vi "VP_Host_Test.vi"() -> ()   [LabVIEW 2015]
uses:
  UI states.ctl
  <vilib>/WebDAVClient/Advanced/Get File.vi
  <vilib>/Utility/config.llb/Write Key (Boolean).vi
  <vilib>/WebDAVClient/Advanced/Put File.vi
  <resource>/objmgr/ni.dex.rc
  <vilib>/nisyscfg/nisyscfg.lvlib
  <resource>/objmgr/nisysapi.rc
  <vilib>/WebDAVClient/NI_WebDAV.lvlib
  <vilib>/Utility/config.llb/NI_LVConfig.lvlib
panel:
  out "Monitor Status":string
  in  "Turn on startup Apps":bool
  in  "Reconnect cRIO":bool
  out "Primary Disk Free (GB)":dbl format="%#_4g"
  out "Primary Disk Capacity (GB)":dbl format="%#_4g"
  out "Free Virtual Memory (GB)":dbl format="%#_4g"
  out "Total Virtual Memory (GB)":dbl format="%#_4g"
  out "Free Physical Memory (GB)":dbl format="%#_4g"
  out "Total Physical Memory (GB)":dbl format="%#_4g"
  out "cRIO System Status":string
  in  "Reboot cRIO":bool
  in  "Target (localhost)":refnum<k21>="localhost"
  in  "Data Loop Period":u32
  out "Velociprobe cRIO error log":string
  in  "Stop Monitor":bool
  in  "Target IP Address":string="localhost"
  out "XY Ref":cluster{dbl[], dbl[]}[](graph)
  out "Reference and Actual positions":cluster{"t0":dbl, dbl, dbl[][]}(graph)
  out "Data Read Period (sec)":dbl=3.9999999999999996e-05
  out "Data Read Rate (Hz)":dbl=25000.000000000004
  out "File plotter loop iterations":i32
  out "Queue is empty":bool=TRUE
  out "Data Frequency":fxp<+,32,0>
  out "Available Elements to Read":i32
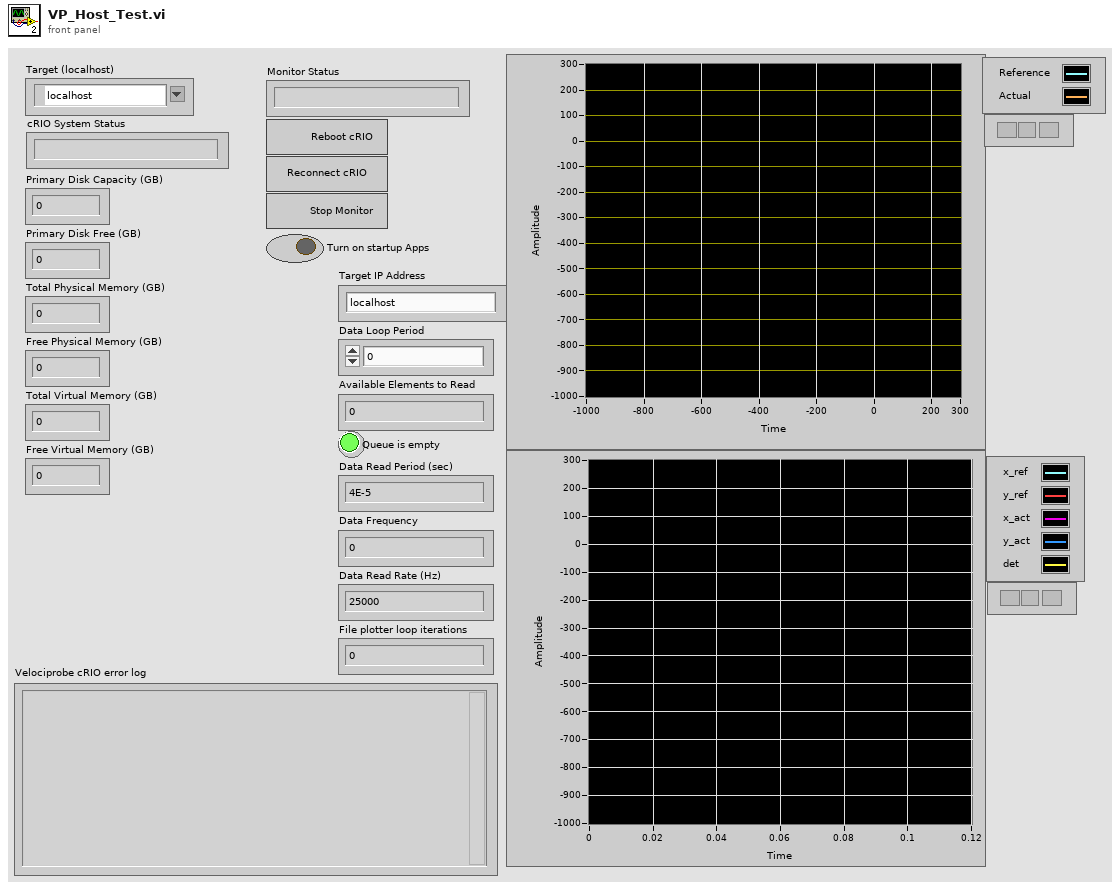
[diagram p1: front panel]
types:
  T1 = typedef "UI states.ctl" = enum16{"Initialize", "Wait", "Turn off cRIO controls "}
  T2 = typedef "NI_WebDAV.lvlib/SessionHandle.ctl" = refnum<k1>
  T3 = typedef "NI_LVConfig.lvlib/Config Data RefNum.ctl" = refnum<k1>
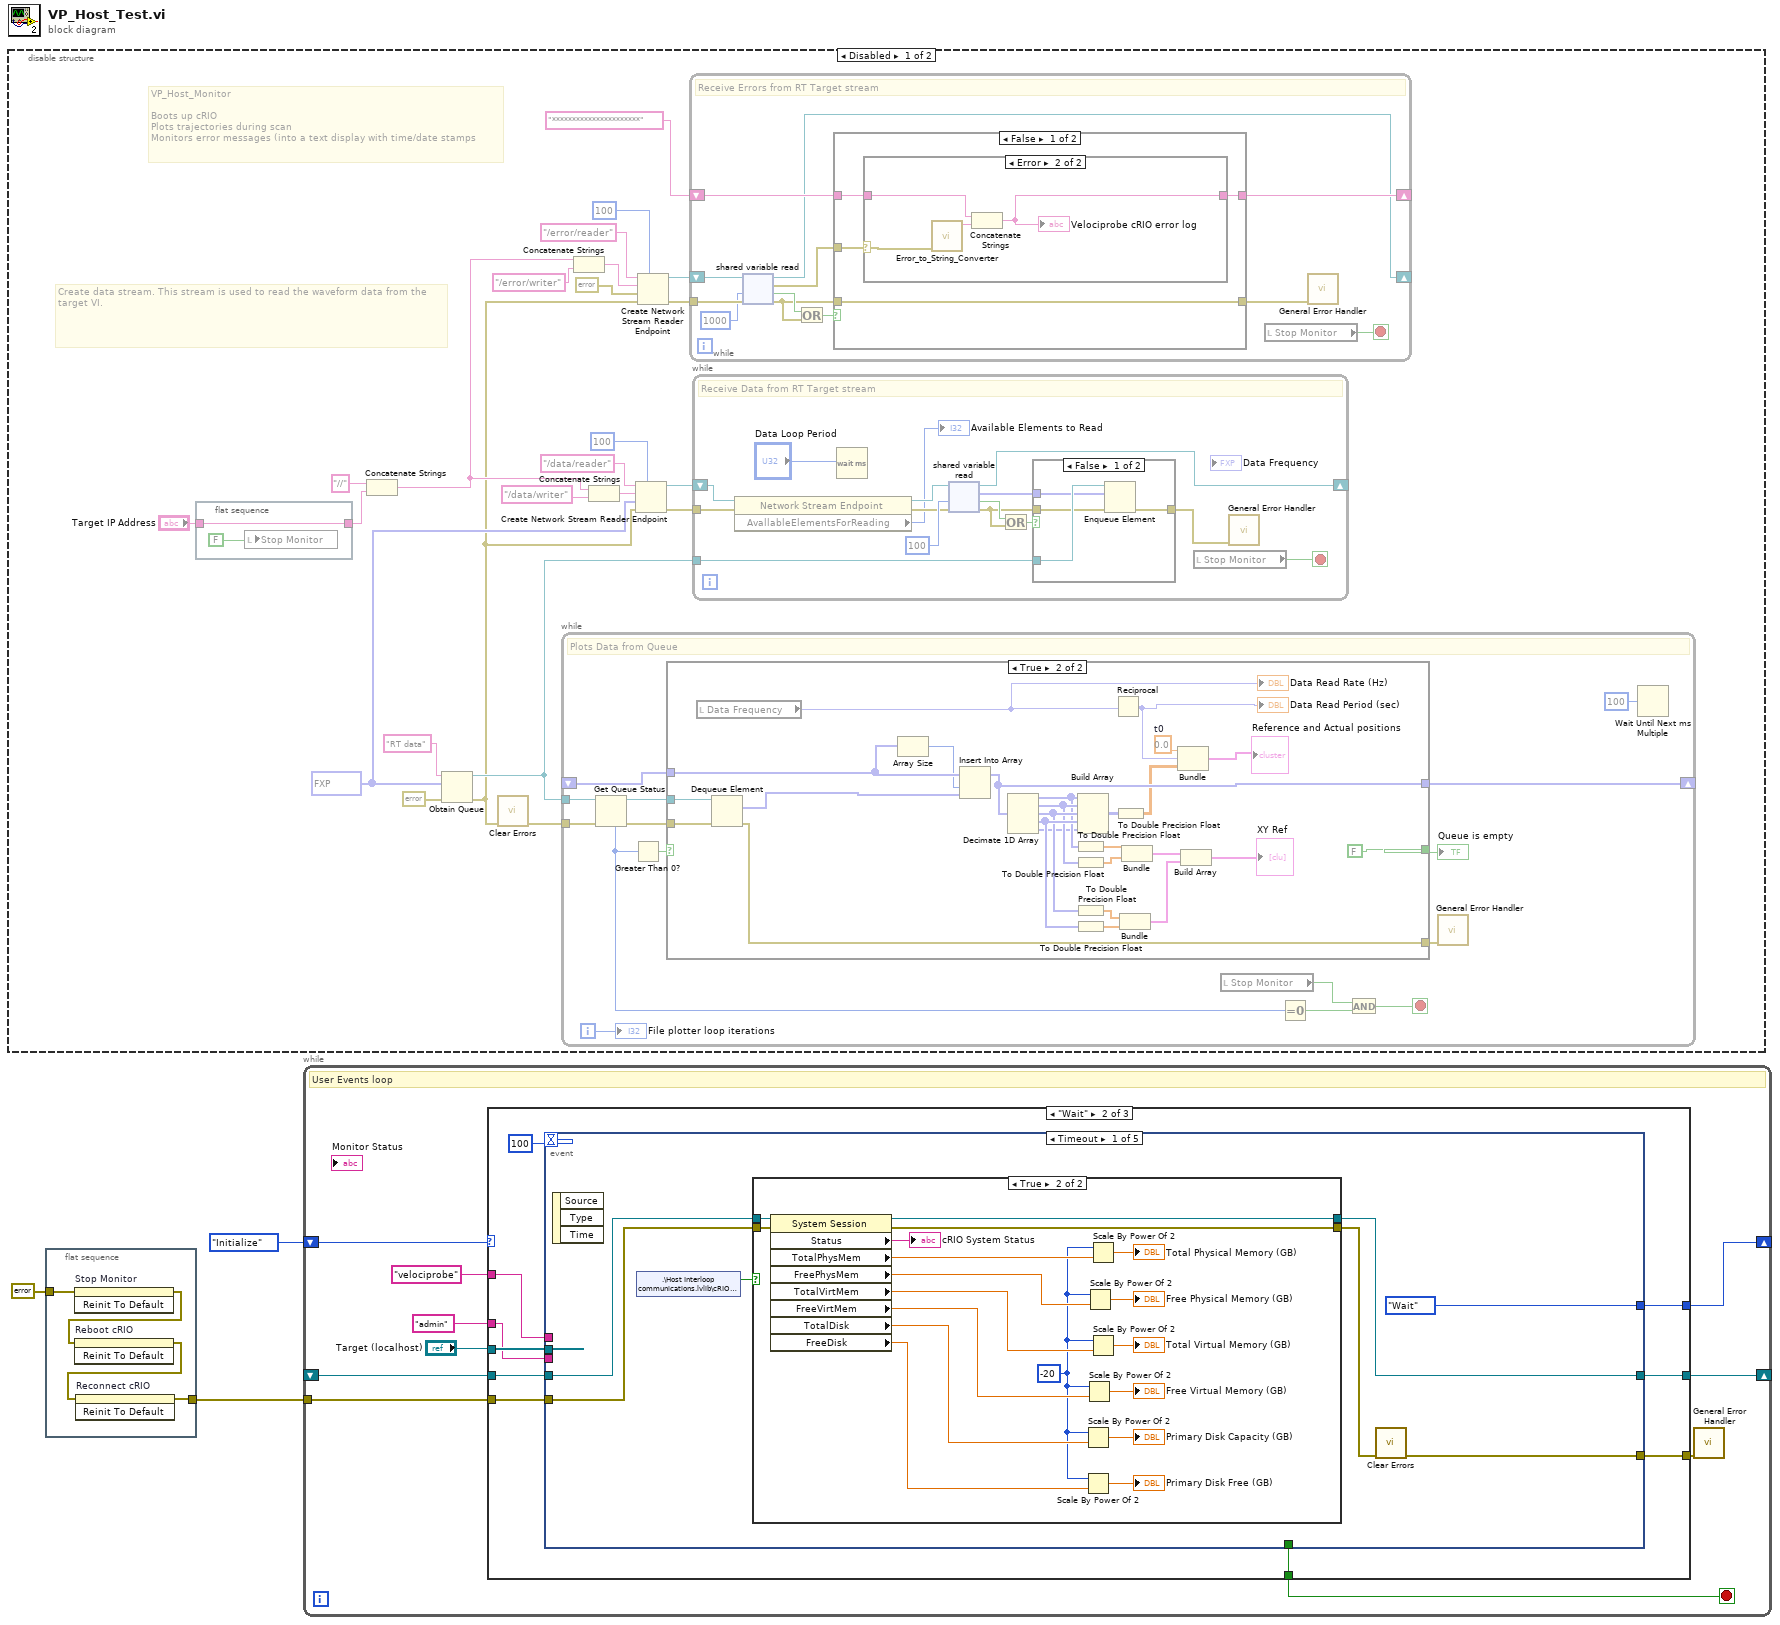
[diagram p0: block diagram]
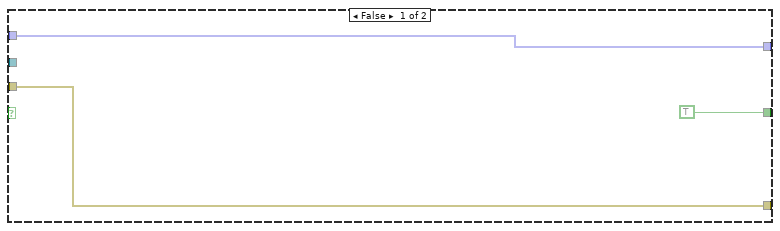
[diagram p4: hidden frame]
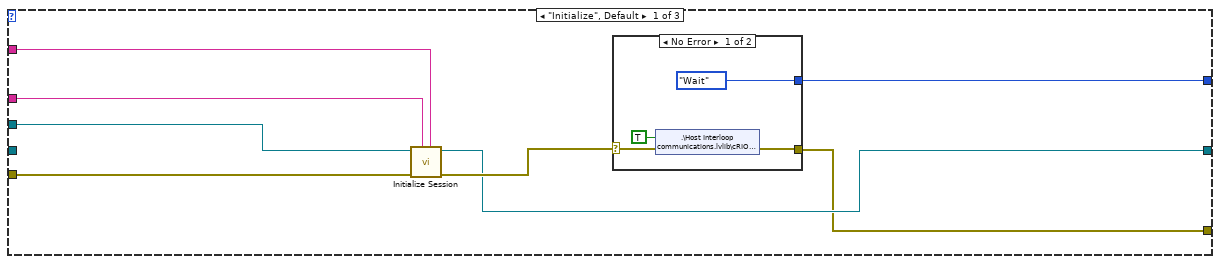
[diagram p7: hidden frame]
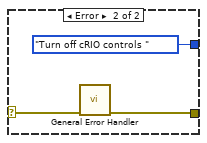
[diagram p8: hidden frame]
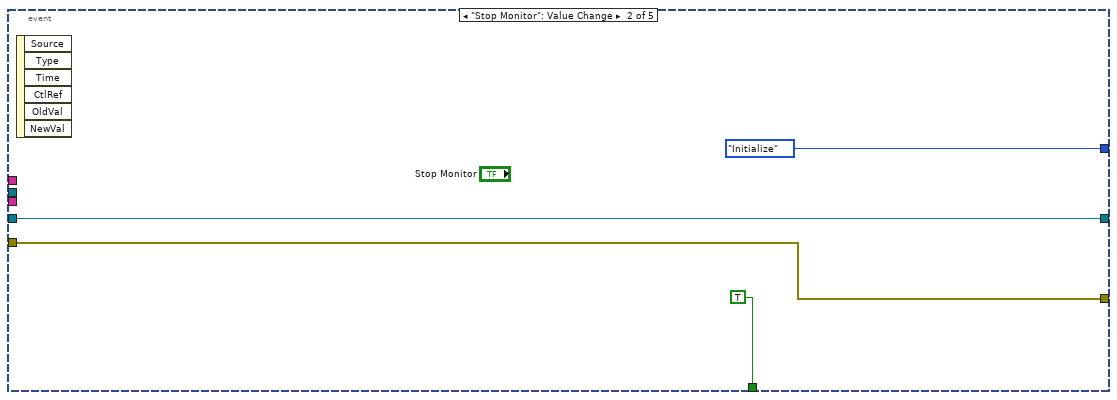
[diagram p10: hidden frame]
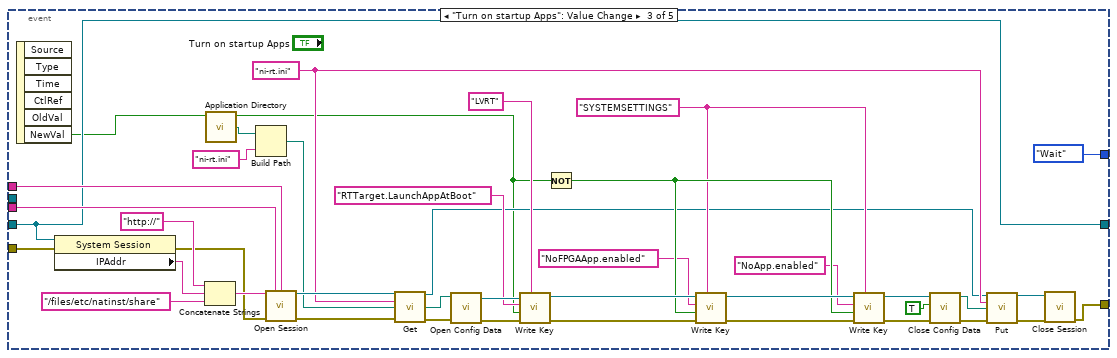
[diagram p11: hidden frame]
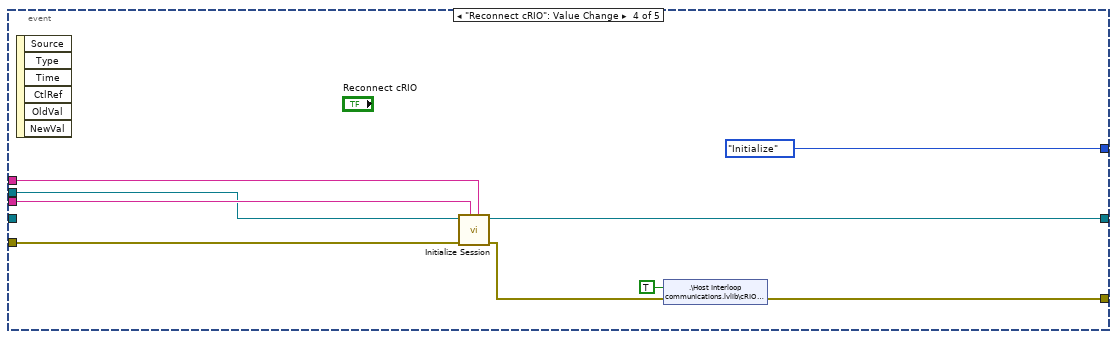
[diagram p12: hidden frame]
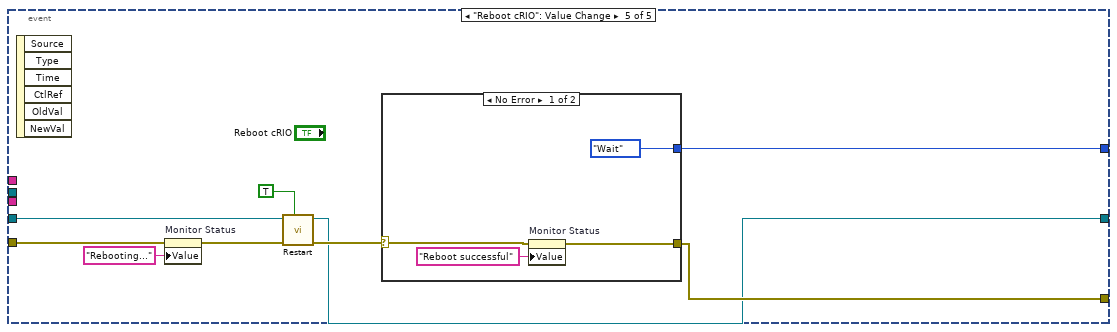
[diagram p13: hidden frame]
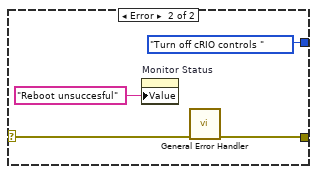
[diagram p14: hidden frame]
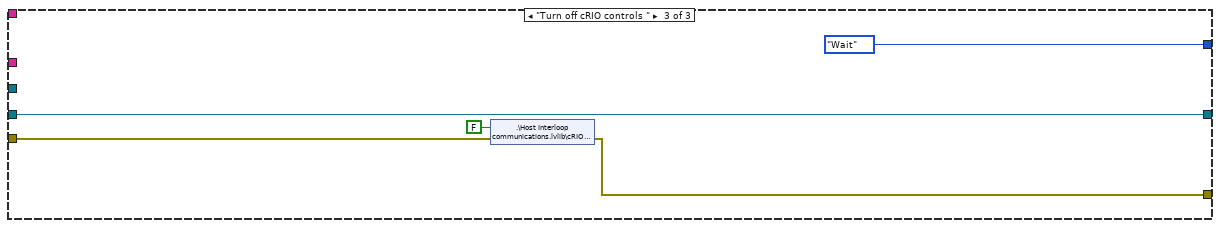
[diagram p15: hidden frame]
diagram:
  n1 = disable-structure shown="Disabled" {
    frame Disabled {
      w16 = fxp<+/-,58,25>[] [0.0, 0.0, 0.0, 0.0, 0.0, 0.0, 0.0, 0.0, 0.0, 0.0, 0.0, 0.0, 0.0, 0.0, 0.0, 0.0, 0.0, 0.0, 0.0, 0.0, 0.0, 0.0, 0.0, 0.0, 0.0, 0.0, 0.0, 0.0, 0.0, 0.0, 0.0, 0.0, 0.0, 0.0, 0.0, 0.0, 0.0, 0.0, 0.0, 0.0, 0.0, 0.0, 0.0, 0.0, 0.0, 0.0, 0.0, 0.0, 0.0, 0.0, 0.0, 0.0, 0.0, 0.0, 0.0, 0.0, 0.0, 0.0, 0.0, 0.0, 0.0, 0.0, 0.0, 0.0, 0.0, 0.0, 0.0, 0.0, 0.0, 0.0, 0.0, 0.0, 0.0, 0.0, 0.0, 0.0, 0.0, 0.0, 0.0, 0.0, 0.0, 0.0, 0.0, 0.0, 0.0, 0.0, 0.0, 0.0, 0.0, 0.0, 0.0, 0.0, 0.0, 0.0, 0.0, 0.0, 0.0, 0.0, 0.0, 0.0, 0.0, 0.0, 0.0, 0.0, 0.0, 0.0, 0.0, 0.0, 0.0, 0.0, 0.0, 0.0, 0.0, 0.0, 0.0, 0.0, 0.0, 0.0, 0.0, 0.0, 0.0, 0.0, 0.0, 0.0, 0.0, 0.0, 0.0, 0.0, 0.0, 0.0, 0.0, 0.0, 0.0, 0.0, 0.0, 0.0, 0.0, 0.0, 0.0, 0.0, 0.0, 0.0, 0.0, 0.0, 0.0, 0.0, 0.0, 0.0, 0.0, 0.0, 0.0, 0.0, 0.0, 0.0, 0.0, 0.0, 0.0, 0.0, 0.0, 0.0, 0.0, 0.0, 0.0, 0.0, 0.0, 0.0, 0.0, 0.0, 0.0, 0.0, 0.0, 0.0, 0.0, 0.0, 0.0, 0.0, 0.0, 0.0, 0.0, 0.0, 0.0, 0.0, 0.0, 0.0, 0.0, 0.0, 0.0, 0.0, 0.0, 0.0, 0.0, 0.0, 0.0, 0.0, 0.0, 0.0, 0.0, 0.0, 0.0, 0.0, 0.0, 0.0, 0.0, 0.0, 0.0, 0.0, 0.0, 0.0, 0.0, 0.0, 0.0, 0.0, 0.0, 0.0, 0.0, 0.0, 0.0, 0.0, 0.0, 0.0, 0.0, 0.0, 0.0, 0.0, 0.0, 0.0, 0.0, 0.0, 0.0, 0.0, 0.0, 0.0, 0.0, 0.0, 0.0, 0.0, 0.0, 0.0, 0.0, 0.0, 0.0, 0.0, 0.0, 0.0, 0.0, 0.0, 0.0, 0.0, 0.0, 0.0, 0.0, 0.0, 0.0, 0.0, 0.0, 0.0, 0.0, 0.0, 0.0, 0.0, 0.0, 0.0, 0.0, 0.0, 0.0, 0.0, 0.0, 0.0, 0.0, 0.0, 0.0, 0.0, 0.0, 0.0, 0.0, 0.0, 0.0, 0.0, 0.0, 0.0, 0.0, 0.0, 0.0, 0.0, 0.0, 0.0, 0.0, 0.0, 0.0, 0.0, 0.0, 0.0, 0.0, 0.0, 0.0, 0.0, 0.0, 0.0, 0.0, 0.0, 0.0, 0.0, 0.0, 0.0, 0.0, 0.0, 0.0, 0.0, 0.0, 0.0, 0.0, 0.0, 0.0, 0.0, 0.0, 0.0, 0.0, 0.0, 0.0, 0.0, 0.0, 0.0, 0.0, 0.0, 0.0, 0.0, 0.0, 0.0, 0.0, 0.0, 0.0, 0.0, 0.0, 0.0, 0.0, 0.0, 0.0, 0.0, 0.0, 0.0, 0.0, 0.0, 0.0, 0.0, 0.0, 0.0, 0.0, 0.0, 0.0, 0.0, 0.0, 0.0, 0.0, 0.0, 0.0, 0.0, 0.0, 0.0, 0.0, 0.0, 0.0, 0.0, 0.0, 0.0, 0.0, 0.0, 0.0, 0.0, 0.0, 0.0, 0.0, 0.0, 0.0, 0.0, 0.0, 0.0, 0.0, 0.0, 0.0, 0.0, 0.0, 0.0, 0.0, 0.0, 0.0, 0.0, 0.0, 0.0, 0.0, 0.0, 0.0, 0.0, 0.0, 0.0, 0.0, 0.0, 0.0, 0.0, 0.0, 0.0, 0.0, 0.0, 0.0, 0.0, 0.0, 0.0, 0.0, 0.0, 0.0, 0.0, 0.0, 0.0, 0.0, 0.0, 0.0, 0.0, 0.0, 0.0, 0.0, 0.0, 0.0, 0.0, 0.0, 0.0, 0.0, 0.0, 0.0, 0.0, 0.0, 0.0, 0.0, 0.0, 0.0, 0.0, 0.0, 0.0, 0.0, 0.0, 0.0, 0.0, 0.0, 0.0, 0.0, 0.0, 0.0, 0.0, 0.0, 0.0, 0.0, 0.0, 0.0, 0.0, 0.0, 0.0, 0.0, 0.0, 0.0, 0.0, 0.0, 0.0, 0.0, 0.0, 0.0, 0.0, 0.0, 0.0, 0.0, 0.0, 0.0, 0.0, 0.0, 0.0, 0.0, 0.0, 0.0, 0.0, 0.0, 0.0, 0.0, 0.0, 0.0, 0.0, 0.0, 0.0, 0.0, 0.0, 0.0, 0.0, 0.0, 0.0, 0.0, 0.0, 0.0, 0.0, 0.0, 0.0, 0.0, 0.0, 0.0, 0.0, 0.0, 0.0, 0.0, 0.0, 0.0, 0.0, 0.0, 0.0, 0.0, 0.0, 0.0, 0.0, 0.0, 0.0, 0.0, 0.0, 0.0, 0.0, 0.0, 0.0, 0.0, 0.0, 0.0, 0.0, 0.0, 0.0, 0.0, 0.0, 0.0, 0.0, 0.0, 0.0, 0.0, 0.0, 0.0, 0.0, 0.0, 0.0, 0.0, 0.0, 0.0, 0.0, 0.0, 0.0, 0.0, 0.0, 0.0, 0.0, 0.0, 0.0, 0.0, 0.0, 0.0, 0.0, 0.0, 0.0, 0.0, 0.0, 0.0, 0.0, 0.0, 0.0, 0.0, 0.0, 0.0, 0.0, 0.0, 0.0, 0.0, 0.0, 0.0, 0.0, 0.0, 0.0, 0.0, 0.0, 0.0, 0.0, 0.0, 0.0, 0.0, 0.0, 0.0, 0.0, 0.0, 0.0, 0.0, 0.0, 0.0, 0.0, 0.0, 0.0, 0.0, 0.0, 0.0, 0.0, 0.0, 0.0, 0.0, 0.0, 0.0, 0.0, 0.0, 0.0, 0.0, 0.0, 0.0, 0.0, 0.0, 0.0, 0.0, 0.0, 0.0, 0.0, 0.0, 0.0, 0.0, 0.0, 0.0, 0.0, 0.0, 0.0, 0.0, 0.0, 0.0, 0.0, 0.0, 0.0, 0.0, 0.0, 0.0, 0.0, 0.0, 0.0, 0.0, 0.0, 0.0, 0.0, 0.0, 0.0, 0.0, 0.0, 0.0, 0.0, 0.0, 0.0, 0.0, 0.0, 0.0, 0.0, 0.0, 0.0, 0.0, 0.0, 0.0, 0.0, 0.0, 0.0, 0.0, 0.0, 0.0, 0.0, 0.0, 0.0, 0.0, 0.0, 0.0, 0.0, 0.0, 0.0, 0.0, 0.0, 0.0, 0.0, 0.0, 0.0, 0.0, 0.0, 0.0, 0.0, 0.0, 0.0, 0.0, 0.0, 0.0, 0.0, 0.0, 0.0, 0.0, 0.0, 0.0, 0.0, 0.0, 0.0, 0.0, 0.0, 0.0, 0.0, 0.0, 0.0, 0.0, 0.0, 0.0, 0.0, 0.0, 0.0, 0.0, 0.0, 0.0, 0.0, 0.0, 0.0, 0.0, 0.0, 0.0, 0.0, 0.0, 0.0, 0.0, 0.0, 0.0, 0.0, 0.0, 0.0, 0.0, 0.0, 0.0, 0.0, 0.0, 0.0, 0.0, 0.0, 0.0, 0.0, 0.0, 0.0, 0.0, 0.0, 0.0, 0.0, 0.0, 0.0, 0.0, 0.0, 0.0, 0.0, 0.0, 0.0, 0.0, 0.0, 0.0, 0.0, 0.0, 0.0, 0.0, 0.0, 0.0, 0.0, 0.0, 0.0, 0.0, 0.0, 0.0, 0.0, 0.0, 0.0, 0.0, 0.0, 0.0, 0.0, 0.0, 0.0, 0.0, 0.0, 0.0, 0.0, 0.0, 0.0, 0.0, 0.0, 0.0, 0.0, 0.0, 0.0, 0.0, 0.0, 0.0, 0.0, 0.0, 0.0, 0.0, 0.0, 0.0, 0.0, 0.0, 0.0, 0.0, 0.0, 0.0, 0.0, 0.0, 0.0, 0.0, 0.0, 0.0, 0.0, 0.0, 0.0, 0.0, 0.0, 0.0, 0.0, 0.0, 0.0, 0.0, 0.0, 0.0, 0.0, 0.0, 0.0, 0.0, 0.0, 0.0, 0.0, 0.0, 0.0, 0.0, 0.0, 0.0, 0.0, 0.0, 0.0, 0.0, 0.0, 0.0, 0.0, 0.0, 0.0, 0.0, 0.0, 0.0, 0.0, 0.0, 0.0, 0.0, 0.0, 0.0, 0.0, 0.0, 0.0, 0.0, 0.0, 0.0, 0.0, 0.0, 0.0, 0.0, 0.0, 0.0, 0.0, 0.0, 0.0, 0.0, 0.0, 0.0, 0.0, 0.0, 0.0, 0.0, 0.0, 0.0, 0.0, 0.0, 0.0, 0.0, 0.0, 0.0, 0.0, 0.0, 0.0, 0.0, 0.0, 0.0, 0.0, 0.0, 0.0, 0.0, 0.0, 0.0, 0.0, 0.0, 0.0, 0.0, 0.0, 0.0, 0.0, 0.0, 0.0, 0.0, 0.0, 0.0, 0.0, 0.0, 0.0, 0.0, 0.0, 0.0, 0.0, 0.0, 0.0, 0.0, 0.0, 0.0, 0.0, 0.0, 0.0, 0.0, 0.0, 0.0, 0.0, 0.0, 0.0, 0.0, 0.0, 0.0, 0.0, 0.0, 0.0, 0.0, 0.0, 0.0, 0.0, 0.0, 0.0, 0.0, 0.0, 0.0, 0.0, 0.0, 0.0, 0.0, 0.0, 0.0, 0.0, 0.0, 0.0, 0.0, 0.0, 0.0, 0.0, 0.0, 0.0, 0.0, 0.0, 0.0, 0.0, 0.0, 0.0, 0.0, 0.0, 0.0, 0.0, 0.0, 0.0, 0.0, 0.0, 0.0, 0.0, 0.0, 0.0, 0.0, 0.0, 0.0, 0.0, 0.0, 0.0, 0.0, 0.0, 0.0, 0.0, 0.0, 0.0, 0.0, 0.0, 0.0, 0.0, 0.0, 0.0, 0.0, 0.0, 0.0, 0.0, 0.0, 0.0, 0.0, 0.0, 0.0, 0.0, 0.0, 0.0, 0.0, 0.0, 0.0, 0.0, 0.0, 0.0, 0.0, 0.0, 0.0, 0.0, 0.0, 0.0, 0.0, 0.0, 0.0, 0.0, 0.0, 0.0, 0.0, 0.0, 0.0, 0.0, 0.0, 0.0, 0.0, 0.0, 0.0, 0.0, 0.0, 0.0, 0.0, 0.0, 0.0, 0.0, 0.0, 0.0, 0.0, 0.0, 0.0, 0.0, 0.0, 0.0, 0.0, 0.0, 0.0, 0.0, 0.0, 0.0, 0.0, 0.0, 0.0, 0.0, 0.0, 0.0, 0.0, 0.0, 0.0, 0.0, 0.0, 0.0, 0.0, 0.0, 0.0, 0.0, 0.0, 0.0, 0.0, 0.0, 0.0, 0.0, 0.0, 0.0, 0.0, 0.0, 0.0, 0.0, 0.0, 0.0, 0.0, 0.0, 0.0, 0.0, 0.0, 0.0, 0.0, 0.0, 0.0, 0.0, 0.0, 0.0, 0.0, 0.0, 0.0, 0.0, 0.0, 0.0, 0.0, 0.0, 0.0, 0.0, 0.0, 0.0, 0.0, 0.0, 0.0, 0.0, 0.0, 0.0, 0.0, 0.0, 0.0, 0.0, 0.0, 0.0, 0.0, 0.0, 0.0, 0.0, 0.0, 0.0, 0.0, 0.0, 0.0, 0.0, 0.0, 0.0, 0.0, 0.0, 0.0, 0.0, 0.0, 0.0, 0.0, 0.0, 0.0, 0.0, 0.0, 0.0, 0.0, 0.0, 0.0, 0.0, 0.0, 0.0, 0.0, 0.0, 0.0, 0.0, 0.0, 0.0, 0.0, 0.0, 0.0, 0.0, 0.0, 0.0, 0.0, 0.0, 0.0, 0.0, 0.0, 0.0, 0.0, 0.0, 0.0, 0.0, 0.0, 0.0, 0.0, 0.0, 0.0, 0.0, 0.0, 0.0, 0.0, 0.0, 0.0, 0.0, 0.0, 0.0, 0.0, 0.0, 0.0, 0.0, 0.0, 0.0, 0.0, 0.0, 0.0, 0.0, 0.0, 0.0, 0.0, 0.0, 0.0, 0.0, 0.0, 0.0, 0.0, 0.0, 0.0, 0.0, 0.0, 0.0, 0.0, 0.0, 0.0, 0.0, 0.0, 0.0, 0.0, 0.0, 0.0, 0.0, 0.0, 0.0, 0.0, 0.0, 0.0, 0.0, 0.0, 0.0, 0.0, 0.0, 0.0, 0.0, 0.0, 0.0, 0.0, 0.0, 0.0, 0.0, 0.0, 0.0, 0.0, 0.0, 0.0, 0.0, 0.0, 0.0, 0.0, 0.0, 0.0, 0.0, 0.0, 0.0, 0.0, 0.0, 0.0, 0.0] ("Data 2")
      # "VP_Host_Monitor\n\nBoots up cRIO\nPlots trajectories during scan\nMonitors error messages (into a text display with time/date stamps"
      # "Create data stream. This stream is used to read the waveform data from the target VI."
      n2 = flat-sequence {
        tunnel: "Target IP Address" -> [w52]
        tunnel: [w52] -> w17
        frame #0 {
          n3 = local write "Stop Monitor"(FALSE ("Host Stop")) -> ()
        }
      }
      n4 = Concatenate Strings("//" ("reader url"), w17) -> (w10:string)
      n5 = Obtain Queue(name (unnamed)="RT data", element data type=w16, error in (no error)=errorcluster {"status"=FALSE, "code"=0, "source"=""}) -> (queue out=w26:refnum<queue>, error out=w8:errorcluster)  [unwired: 2 in, 1 out]
      n6 = call <vilib>:"Clear Errors.vi"("error in (no error)"=w8) -> ("error out"=w27:errorcluster)  [unwired: 5 in, 1 out]
      n7 = while {
        tunnel: w26 -> [w67]
        shift-right: [w57] -> _
        shift-left: _ -> [w56]
        tunnel: w27 -> [w66]
        i -> [w59]
        stop <- w60 stop-if-true
        # "Plots Data from Queue"
        n8 = Get Queue Status(queue=w67, error in (no error)=w66) -> (queue out=w64:refnum<queue>, error out=w65:errorcluster, # elements in queue=w62:i32)  [unwired: 1 in, 5 out]
        n9 = Greater Than 0?(x=w62) -> (x > 0?=w63:bool)
        n10 = case shown="True" w63 {
          tunnel: w65 -> [w69 w96]
          tunnel: w64 -> [_ w95]
          tunnel: [w69 w86] -> w53
          tunnel: [TRUE FALSE] -> w58
          tunnel: [w68 w93] -> w57
          tunnel: w56 -> [w68 w92]
          frame False {
          }
          frame True {
            w79 = 0.0  # t0
            n11 = local read "Data Frequency"() -> (w87:fxp<+,32,0>)
            "Data Read Rate (Hz)" <- w87
            n12 = Dequeue Element(queue=w95, error in (no error)=w96) -> (element=w91:fxp<+/-,58,25>[], error out=w86:errorcluster)  [unwired: 1 in, 2 out]
            n13 = Array Size(array=w92) -> (size(s)=w73:i32)
            n14 = Insert Into Array(array=w92, index=w73, new element=w91) -> (w93:fxp<+/-,58,25>[])
            n15 = Decimate 1D Array(w93) -> (w82:fxp<+/-,58,25>[], w83:fxp<+/-,58,25>[], w84:fxp<+/-,58,25>[], w85:fxp<+/-,58,25>[], w81:fxp<+/-,58,25>[])
            n16 = To Double Precision Float(number=w82) -> (double precision float=w77:dbl[])
            n17 = To Double Precision Float(number=w83) -> (double precision float=w76:dbl[])
            n18 = To Double Precision Float(number=w84) -> (double precision float=w75:dbl[])
            n19 = To Double Precision Float(number=w85) -> (double precision float=w74:dbl[])
            n20 = Build Array(w82, w83, w84, w85, w81) -> (w80:fxp<+/-,58,25>[][])
            n21 = Reciprocal(x=w87) -> (1/x=w88:fxp<+,33,33>)
            "Data Read Period (sec)" <- w88
            n22 = To Double Precision Float(number=w80) -> (double precision float=w71:dbl[][])
            n23 = Bundle(w75, w74) -> (w72:cluster{dbl[], dbl[]})  [unwired: 1 in]
            n24 = Bundle(w77, w76) -> (w78:cluster{dbl[], dbl[]})  [unwired: 1 in]
            n25 = Bundle("t0"=w79, w88, w71) -> (→"Reference and Actual positions":cluster{"t0":dbl, fxp<+,33,33>, dbl[][]})  [unwired: 1 in]
            n26 = Build Array(w78, w72) -> (→"XY Ref":cluster{dbl[], dbl[]}[])
          }
        }
        "Queue is empty" <- w58
        n27 = local read "Stop Monitor"() -> (w54:bool)
        n28 = Equal To 0?(x=w62) -> (x = 0?=w61:bool)
        n29 = And(x=w54, y=w61) -> (x .and. y?=w60:bool)
        n30 = call <vilib>:"General Error Handler.vi"("error in (no error)"=w53) -> ()  [unwired: 10 in, 5 out]
        n31 = Wait Until Next ms Multiple(millisecond multiple=u32 100) -> ()  [unwired: 1 out]
        "File plotter loop iterations" <- w59
      }
      n32 = Concatenate Strings(w10, "/error/writer" ("reader url")) -> (w13:string)
      n33 = Concatenate Strings(w10, "/data/writer" ("reader url")) -> (w20:string)
      n34 = Create Network Stream Reader Endpoint(7:100 ("reader buffer size"), 8:w8, 9:w16, 10:w20, 11:"/data/reader" ("writer name")) -> (0:w9:errorcluster, 3:w15:refnum<k21>)  [unwired: 2 in]
      n35 = Create Network Stream Reader Endpoint(7:100 ("reader buffer size"), 8:w8, 9:errorcluster {"status"=FALSE, "code"=0, "source"=""} ("error constant"), 10:w13, 11:"/error/reader" ("writer name")) -> (0:w5:errorcluster, 3:w6:refnum<k21>)  [unwired: 2 in]
      n36 = while "Host->Target Command Reader" {
        shift-right: [w29] -> _
        shift-left: w6 -> [w38]
        shift-right: [w31] -> _
        shift-left: "**********************" -> [w30]
        tunnel: w5 -> [w39]
        stop <- w32 stop-if-true
        # "Receive Errors from RT Target stream"
        n37 = shared-variable-read(w38, w39, 1000 ("timeout ms")) -> (w29:refnum<k21>, w33:errorcluster, w35:bool, w36:errorcluster)
        n38 = Or(x=w35, y=w33) -> (x .or. y?=w34:bool)
        n39 = case shown="False" w34 {
          tunnel: w33 -> [w43 w50]
          tunnel: [w43 w50] -> w28
          tunnel: w36 -> [w40 _]
          tunnel: [w42 w49] -> w31
          tunnel: w30 -> [w41 w49]
          frame False {
            n40 = case shown="Error" w40 {
              selector: w40 -> [_ w48]
              tunnel: [w44 w46] -> w42
              tunnel: w41 -> [w44 w45]
              frame No Error {
              }
              frame Error {
                n41 = call "Error_to_String_Converter.vi"("error in"=w48) -> ("String"=w47:string)  [unwired: 9 in, 1 out]
                n42 = Concatenate Strings(w45, w47) -> (w46:string)
                "Velociprobe cRIO error log" <- w46
              }
            }
          }
          frame True {
          }
        }
        n43 = local read "Stop Monitor"() -> (w32:bool)
        n44 = call <vilib>:"General Error Handler.vi"("error in (no error)"=w28) -> ()  [unwired: 10 in, 5 out]
      }
      n45 = while "Target->Host Data Reader" {
        shift-right: [w108] -> _
        shift-left: w15 -> [w105]
        tunnel: w26 -> [w100]
        tunnel: w9 -> [w103]
        stop <- w99 stop-if-true
        # "Receive Data from RT Target stream"
        n46 = property class="Network Stream Endpoint"(reference=w105, error in=w103) -> (reference out=w104:refnum<k21>, error out=w102:errorcluster, "AvallableElementsForReading"=→"Available Elements to Read":i32)
        n47 = Wait (ms)(milliseconds to wait="Data Loop Period") -> ()  [unwired: 1 out]
        n48 = shared-variable-read(w104, w102, 100 ("timeout ms")) -> (w108:refnum<k21>, w107:errorcluster, w110:bool, w111:fxp<+/-,58,25>[])
        n49 = Or(x=w110, y=w107) -> (x .or. y?=w109:bool)
        n50 = case shown="False" w109 {
          tunnel: w111 -> [w114 _]
          tunnel: w107 -> [w113 w116]
          tunnel: [w112 w116] -> w97
          tunnel: w100 -> [w115 _]
          frame False {
            n51 = Enqueue Element(queue=w115, element=w114, error in (no error)=w113) -> (error out=w112:errorcluster)  [unwired: 1 in, 2 out]
          }
          frame True {
          }
        }
        n52 = local read "Stop Monitor"() -> (w99:bool)
        n53 = call <vilib>:"General Error Handler.vi"("error in (no error)"=w97) -> ()  [unwired: 10 in, 5 out]
      }
    }
    frame Enabled {
    }
  }
  n54 = flat-sequence {
    tunnel: errorcluster {"status"=FALSE, "code"=0, "source"=""} ("error in (no error)") -> [w118]
    tunnel: [w117] -> w1
    frame #0 {
      n55 = invoke on="Stop Monitor" class="Bool" method="Reinit To Default"(error in=w118) -> (error out=w120:errorcluster)  [unwired: 2 in, 2 out]
      n56 = invoke on="Reboot cRIO" class="Bool" method="Reinit To Default"(error in=w120) -> (error out=w119:errorcluster)  [unwired: 2 in, 2 out]
      n57 = invoke on="Reconnect cRIO" class="Bool" method="Reinit To Default"(error in=w119) -> (error out=w117:errorcluster)  [unwired: 2 in, 2 out]
    }
  }
  n58 = while {
    tunnel: w1 -> [w128]
    shift-right: [w126] -> _
    shift-left: UI_states."Initialize" -> [w127]
    shift-right: [w125] -> _
    shift-left: _ -> [w129]
    stop <- w130 stop-if-true
    # "User Events loop"
    n59 = case shown="\"Wait\"" w127 {
      tunnel: [_ w155 _] -> w130
      tunnel: w129 -> [_ w153 w253]
      tunnel: w128 -> [w136 w152 w254]
      tunnel: [w135 w151 UI_states."Wait"] -> w126
      tunnel: [w137 w149 w253] -> w125
      tunnel: [w134 w150 w255] -> w124
      tunnel: "Target (localhost)" -> [w133 w146 _]
      tunnel: "velociprobe" ("Password") -> [w132 w147 _]
      tunnel: "admin" ("User Name") -> [w131 w148 _]
      frame "Initialize", Default {
        n60 = call <vilib>:"Initialize Session.vi"("Password"=w132, "User Name"=w131, "error in (no error)"=w136, "Target (localhost)"=w133) -> ("error out"=w138:errorcluster, "Session out"=w137:refnum<k21>)  [unwired: 6 in]
        n61 = case shown="No Error" w138 {
          selector: w138 -> [w141 w144]
          tunnel: [UI_states."Wait" UI_states."Turn off cRIO controls "] -> w135
          tunnel: [w140 w143] -> w134
          frame No Error {
            n62 = shared-variable ".\\Host Interloop communications.lvlib\\cRIO status"(TRUE ("cRIO status"), error in=w141) -> (error out=w140:errorcluster)
          }
          frame Error {
            n63 = call <vilib>:"General Error Handler.vi"("error in (no error)"=w144) -> ("error out"=w143:errorcluster)  [unwired: 10 in, 4 out]
          }
        }
      }
      frame "Wait" {
        n64 = event shown="[0] Timeout" {
          selector: _ -> [_ _ _ _ _]
          dyn-events: _ -> [_ _ _ _ _]
          timeout: 100 -> [_ _ _ _ _]
          tunnel: [_ TRUE _ _ _] -> w155
          tunnel: w153 -> [w162 w183 w188 _ w244]
          tunnel: w152 -> [w161 w184 w226 w233 w237]
          tunnel: [UI_states."Wait" UI_states."Initialize" UI_states."Wait" UI_states."Initialize" w243] -> w151
          tunnel: [w156 w184 w210 w228 w241] -> w150
          tunnel: [w157 w183 w188 w234 w240] -> w149
          tunnel: w148 -> [_ _ w190 w232 _]
          tunnel: w147 -> [_ _ w189 w231 _]
          tunnel: w146 -> [_ _ _ w230 _]
          event Timeout {
            n65 = event-data() -> ()  [unwired: 1 in, 3 out]
            n66 = shared-variable ".\\Host Interloop communications.lvlib\\cRIO status"() -> (w159:bool)  [unwired: 1 in, 1 out]
            n67 = case shown="True" w159 {
              tunnel: w162 -> [w163 w182]
              tunnel: w161 -> [w164 w181]
              tunnel: [w164 w174] -> w158
              tunnel: [w163 w173] -> w157
              frame False {
              }
              frame True {
                w165 = -20
                n68 = property class="System Session"(reference=w182, error in=w181) -> (reference out=w173:refnum<k21>, error out=w174:errorcluster, "Status"=→"cRIO System Status":string, "TotalPhysMem"=w179:dbl, "FreePhysMem"=w178:dbl, "TotalVirtMem"=w172:dbl, "FreeVirtMem"=w177:dbl, "TotalDisk"=w176:dbl, "FreeDisk"=w175:dbl)
                n69 = Scale By Power Of 2(n=w165, x=w176) -> (x*2^n=→"Primary Disk Capacity (GB)":dbl)
                n70 = Scale By Power Of 2(n=w165, x=w175) -> (x*2^n=→"Primary Disk Free (GB)":dbl)
                n71 = Scale By Power Of 2(n=w165, x=w177) -> (x*2^n=→"Free Virtual Memory (GB)":dbl)
                n72 = Scale By Power Of 2(n=w165, x=w178) -> (x*2^n=→"Free Physical Memory (GB)":dbl)
                n73 = Scale By Power Of 2(n=w165, x=w179) -> (x*2^n=→"Total Physical Memory (GB)":dbl)
                n74 = Scale By Power Of 2(n=w165, x=w172) -> (x*2^n=→"Total Virtual Memory (GB)":dbl)
              }
            }
            n75 = call <vilib>:"Clear Errors.vi"("error in (no error)"=w158) -> ("error out"=w156:errorcluster)  [unwired: 5 in, 1 out]
          }
          event "Stop Monitor": Value Change {
            n76 = event-data() -> ()  [unwired: 1 in, 6 out]
          }
          event "Turn on startup Apps": Value Change {
            w195 = "SYSTEMSETTINGS" ("section")
            w208 = "ni-rt.ini" ("username")
            n77 = event-data() -> ("NewVal"=w187:bool)  [unwired: 1 in, 5 out]
            n78 = property class="System Session"(reference=w188, error in=w226) -> (error out=w221:errorcluster, "IPAddr"=w225:string)  [unwired: 1 out]
            n79 = Concatenate Strings("http://" ("string"), w225, "/files/etc/natinst/share" ("string")) -> (w222:string)
            n80 = call <vilib>:"Application Directory.vi"() -> ("Application Directory"=w216:path)
            n81 = Build Path(base path=w216, name or relative path="ni-rt.ini" ("username")) -> (appended path=w217:path)
            n82 = call <vilib>:"Open Session.vi"("host uri prefix"=w222, "username"=w190, "password"=w189, "error in (no error)"=w221) -> ("session handle out"=w219:T2, "error out"=w220:errorcluster)  [unwired: 10 in]
            n83 = call-poly <vilib>:"Get.vi"("session handle"=w219, "relative uri"=w208, "local file path"=w217, "error in (no error)"=w220) -> ("session handle out"=w192:T2, "local file path out"=w214:path, "error out"=w215:errorcluster)  [unwired: 9 in]
            n84 = call <vilib>:"Open Config Data.vi"("error in (no error)"=w215, "configuration file path"=w214) -> ("error out"=w206:errorcluster, "refnum"=w205:T3)  [unwired: 7 in, 1 out]
            n85 = call-poly <vilib>:"Write Key.vi"("section"="LVRT", "error in (no error)"=w206, "value"=w187, "key"="RTTarget.LaunchAppAtBoot", "refnum"=w205) -> ("error out"=w202:errorcluster, "refnum out"=w199:T3)  [unwired: 4 in, 1 out]
            n86 = Not(x=w187) -> (.not. x?=w196:bool)
            n87 = call-poly <vilib>:"Write Key.vi"("section"=w195, "error in (no error)"=w202, "value"=w196, "key"="NoFPGAApp.enabled", "refnum"=w199) -> ("error out"=w201:errorcluster, "refnum out"=w198:T3)  [unwired: 4 in, 1 out]
            n88 = call-poly <vilib>:"Write Key.vi"("section"=w195, "error in (no error)"=w201, "value"=w196, "key"="NoApp.enabled", "refnum"=w198) -> ("error out"=w200:errorcluster, "refnum out"=w197:T3)  [unwired: 4 in, 1 out]
            n89 = call <vilib>:"Close Config Data.vi"("error in (no error)"=w200, "write file if changed (T)"=TRUE, "refnum"=w197) -> ("error out"=w213:errorcluster, "file path"=w191:path)  [unwired: 7 in]
            n90 = call-poly <vilib>:"Put.vi"("session handle"=w192, "relative uri"=w208, "local file path"=w191, "error in (no error)"=w213) -> ("session handle out"=w212:T2, "error out"=w211:errorcluster)  [unwired: 9 in, 1 out]
            n91 = call <vilib>:"Close Session.vi"("session handle"=w212, "error in (no error)"=w211) -> ("error out"=w210:errorcluster)  [unwired: 13 in]
          }
          event "Reconnect cRIO": Value Change {
            n92 = event-data() -> ()  [unwired: 1 in, 6 out]
            n93 = call <vilib>:"Initialize Session.vi"("Password"=w231, "User Name"=w232, "error in (no error)"=w233, "Target (localhost)"=w230) -> ("error out"=w229:errorcluster, "Session out"=w234:refnum<k21>)  [unwired: 6 in]
            n94 = shared-variable ".\\Host Interloop communications.lvlib\\cRIO status"(TRUE ("cRIO status"), error in=w229) -> (error out=w228:errorcluster)
          }
          event "Reboot cRIO": Value Change {
            n95 = event-data() -> ()  [unwired: 1 in, 6 out]
            n96 = property on="Monitor Status" class="Str"(error in=w237, "Value"="Rebooting..." ("Status")) -> (error out=w238:errorcluster)  [unwired: 1 in, 1 out]
            n97 = call <vilib>:"Restart.vi"("Wait Until Complete (T)"=TRUE, "error in (no error)"=w238, "Session in"=w244) -> ("error out"=w242:errorcluster, "Session out"=w240:refnum<k21>)  [unwired: 6 in, 1 out]
            n98 = case shown="No Error" w242 {
              selector: w242 -> [w246 w251]
              tunnel: [UI_states."Wait" UI_states."Turn off cRIO controls "] -> w243
              tunnel: [w245 w250] -> w241
              frame No Error {
                n99 = property on="Monitor Status" class="Str"(error in=w246, "Value"="Reboot successful" ("Status")) -> (error out=w245:errorcluster)  [unwired: 1 in, 1 out]
              }
              frame Error {
                n100 = property on="Monitor Status" class="Str"("Value"="Reboot unsuccesful" ("Tip Strip")) -> ()  [unwired: 2 in, 2 out]
                n101 = call <vilib>:"General Error Handler.vi"("error in (no error)"=w251) -> ("error out"=w250:errorcluster)  [unwired: 10 in, 4 out]
              }
            }
          }
        }
      }
      frame "Turn off cRIO controls " {
        n102 = shared-variable ".\\Host Interloop communications.lvlib\\cRIO status"(FALSE ("cRIO status"), error in=w254) -> (error out=w255:errorcluster)
      }
    }
    n103 = call <vilib>:"General Error Handler.vi"("error in (no error)"=w124) -> ()  [unwired: 10 in, 5 out]
  }
